vi "Assert 2D Array wired to Scalar Type.vi"   [LabVIEW 2017]
uses:
  ee9912fa-20a1-4971-bda0-633167eee7ad.vi
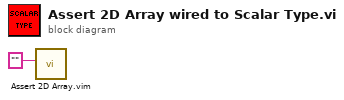
[diagram p0: block diagram]
diagram:
  n1 = call "Assert 2D Array.vim"("Array in"="") -> ()  [unwired: 10 in, 1 out]
